vi "Init.vi"(8 "error in (no error)":errorcluster, 10 "Prevent Cache":bool) -> (0 "error out":errorcluster, 3 "GodotHeaders out":refnum<class "GodotHeaders.lvclass">)   [LabVIEW 2020, in "GodotLV.lvlib" / "GodotHeaders.lvclass"]
uses:
  GodotHeaders.lvclass
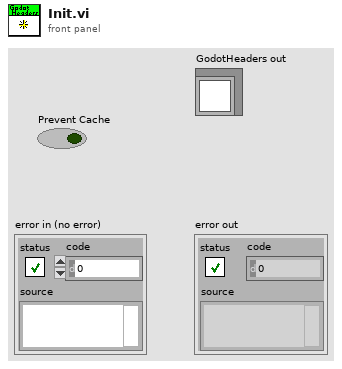
[diagram p1: front panel]
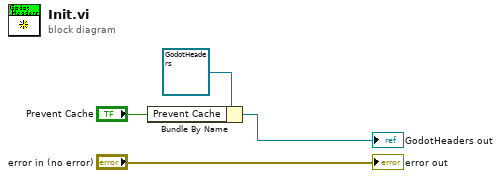
[diagram p0: block diagram]
diagram:
  n1 = Bundle By Name(cluster=refnum<class "GodotHeaders.lvclass"> refnum ("GodotHeaders in"), "Prevent Cache"="Prevent Cache") -> (→"GodotHeaders out":refnum<class "GodotHeaders.lvclass">)
  "error out" <- "error in (no error)"
